vi "Pin to Pin Array.vi"(11 "pin or relay name":string) -> (3 "pin array":string[](array[string]))   [LabVIEW 2020, in "MeasurementLink Session Management.lvlib" / "Session Reservation.lvclass"]
uses:
  Session Reservation.lvclass
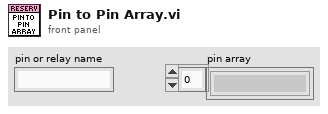
[diagram p1: front panel]
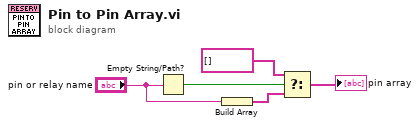
[diagram p0: block diagram]
diagram:
  n1 = Empty String/Path?(string/path="pin or relay name") -> (empty?=w2:bool)
  n2 = Build Array("pin or relay name") -> (w3:string[])
  n3 = Select(t=string[] [], s=w2, f=w3) -> (s? t:f=→"pin array":string[])
